vi "log_raw_data.vi"(8 "error in":errorcluster, 9 "Trace info":T1, 10 "Timestamp":timestamp, 11 "Raw file":refnum<file>) -> (0 "error out":errorcluster, 3 "Raw file out":refnum<file>)   [LabVIEW 2026]
uses:
  gui/trace_info.ctl
  gui/trace_channel.ctl
  main/ilemt_status.ctl
panel:
  # "This is a relative timestamp, zero at startup. It increments deterministically."
  # "Log \"Raw data\" from \"Trace Info\""
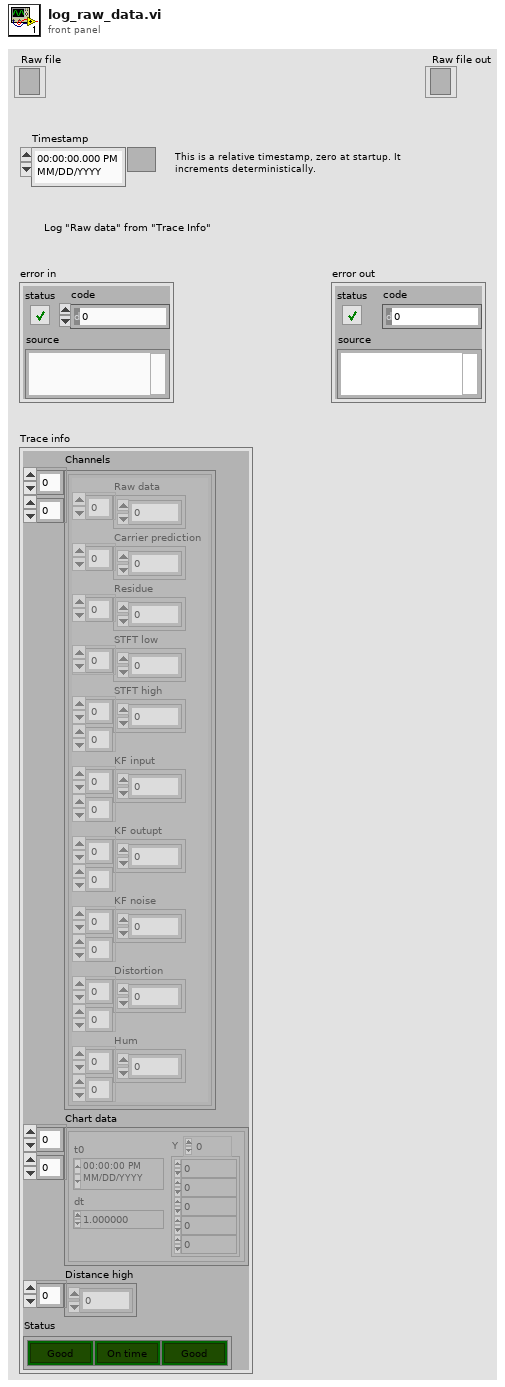
[diagram p1: front panel]
types:
  T1 = typedef "trace_info.ctl" = cluster{"Channels":T2[][], "Chart data":waveform(dbl)[][], "Distance high":dbl[], "Status":T3}
  T2 = typedef "trace_channel.ctl" = cluster{"Raw data":dbl[], "Carrier prediction":dbl[], "Residue":dbl[], "STFT low":cdb[], "STFT high":cdb[][], "KF input":cdb[][], "KF outupt":cdb[][], "KF noise":dbl[][], "Distortion":cdb[][], "Hum":cdb[][]}
  T3 = typedef "ilemt_status.ctl" = cluster{"NaN":bool, "Backlog":bool, "Clipping":bool}
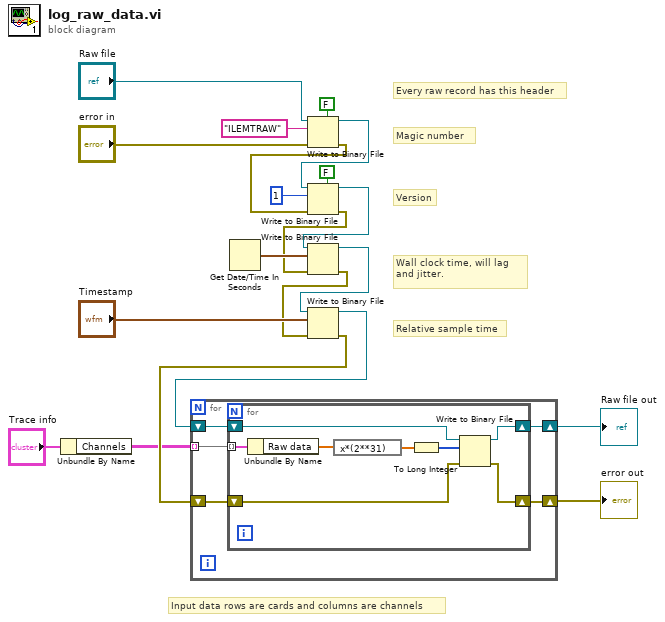
[diagram p0: block diagram]
diagram:
  # "Every raw record has this header"
  # "Relative sample time"
  # "Wall clock time, will lag and jitter."
  # "Version"
  # "Magic number"
  # "Input data rows are cards and columns are channels"
  n1 = Unbundle By Name("Trace info") -> ("Channels"=w1:T2[][])
  n2 = Get Date/Time In Seconds() -> (seconds since 1Jan1904=w16:timestamp)
  n3 = Write to Binary File(file (use dialog)="Raw file", data="ILEMTRAW", error in="error in", 5:FALSE ("prepend array or string size? (T)")) -> (refnum out=w8:refnum<file>, error out=w5:errorcluster)  [unwired: 2 in, 1 out]
  n4 = Write to Binary File(file (use dialog)=w8, data=1, error in=w5, 5:FALSE ("prepend array or string size? (T)")) -> (refnum out=w3:refnum<file>, error out=w6:errorcluster)  [unwired: 2 in, 1 out]
  n5 = Write to Binary File(file (use dialog)=w3, data=w16, error in=w6) -> (refnum out=w15:refnum<file>, error out=w14:errorcluster)  [unwired: 3 in, 1 out]
  n6 = Write to Binary File(file (use dialog)=w15, data="Timestamp", error in=w14) -> (refnum out=w13:refnum<file>, error out=w12:errorcluster)  [unwired: 3 in, 1 out]
  n7 = for {
    tunnel: w1 -> [w25] mode=indexing
    shift-right: [w23] -> w4
    shift-left: w13 -> [w24]
    shift-right: [w21] -> w18
    shift-left: w12 -> [w22]
    n8 = for {
      tunnel: w25 -> [w29] mode=indexing
      shift-right: [w32] -> w23
      shift-left: w24 -> [w33]
      shift-right: [w30] -> w21
      shift-left: w22 -> [w31]
      n9 = Unbundle By Name(w29) -> ("Raw data"=w28:dbl[])
      n10 = expression code="x*(2**31)"(w28) -> (w27:dbl[])
      n11 = To Long Integer(number=w27) -> (32bit integer=w26:i32[])
      n12 = Write to Binary File(file (use dialog)=w33, data=w26, error in=w31) -> (refnum out=w32:refnum<file>, error out=w30:errorcluster)  [unwired: 3 in, 1 out]
    }
  }
  "error out" <- w18
  "Raw file out" <- w4
